vi "eta2cont (SubVI).vi"(11 "eta_disc":dbl[](array[numeric])) -> (2 "count":dbl, 3 "eta_cont":dbl[](array[numeric]))   [LabVIEW 2014]
uses:
  <vilib>/imath/engines/lvmath2/RunTimeEngine/IndexRead/NIMS V(S).vi
  <instcachedir>/0/NIMS V(S)_0488751826AF41519A22953C041130DC.lvgen/NIMS V(S)_0488751826AF41519A22953C041130DC_000.vi
  <vilib>/imathl/engines/lvmath/Functions/Error Handling/Create Error.vi
  <vilib>/imath/engines/lvmath2/RunTimeEngine/IndexReplace/NIMS V(S)=S.vi
  <instcachedir>/0/NIMS V(S)=S_2D52C4EC15D8415E870AEE69FB516CCA.lvgen/NIMS V(S)=S_2D52C4EC15D8415E870AEE69FB516CCA_000.vi
  <vilib>/imath/engines/lvmath2/RunTimeEngine/NodeEndStatement/NIMS_NodeEndStatement_Output.vi
  <instcachedir>/0/NIMS_NodeEndStatement_Output_53EC0D466D134D7ABD903AC30B43404B.lvgen/NIMS_NodeEndStatement_Output_53EC0D466D134D7ABD903AC30B43404B_005.vi
  <instcachedir>/0/NIMS_NodeEndStatement_Output_53EC0D466D134D7ABD903AC30B43404B.lvgen/NIMS_NodeEndStatement_Output_53EC0D466D134D7ABD903AC30B43404B_001.vi
  <vilib>/imath/engines/lvmath2/RunTimeEngine/ErrorHandling/NIMS_Finalize Error.vi
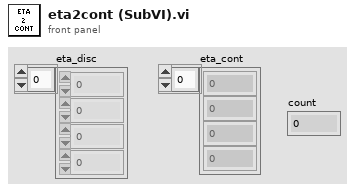
[diagram p1: front panel]
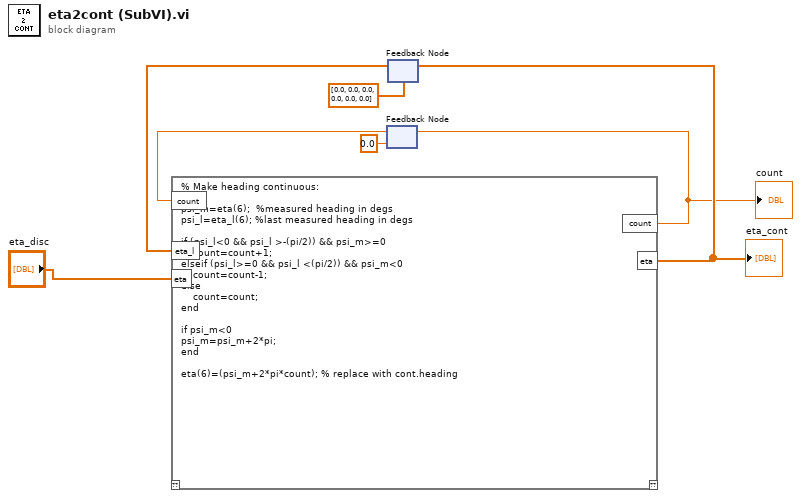
[diagram p0: block diagram]
diagram:
  n1 = feedback #1(0.0 ("count")) -> (w4:dbl)
  n2 = feedback #2(dbl[] [0.0, 0.0, 0.0, 0.0, 0.0, 0.0] ("eta")) -> (w6:dbl[])
  n3 = mathscript code="% Make heading continuous:\n\npsi_m=eta(6);  %measured heading in degs\npsi_l=eta_l(6); %last measured heading in degs\n\nif (psi_l<0 && psi_l >-(pi/2)) && psi_m>=0\n    count=count+1;    \nelseif (psi_l>=0 && psi_l <(pi/2)) && psi_m<0\n    count=count-1;\nelse    \n    count=count;\nend\n\nif psi_m<0\npsi_m=psi_m+2*pi;\nend\n\neta(6)=(psi_m+2*pi*count); % replace with cont.heading"("eta"="eta_disc", "eta_l"=w6, "count"=w4) -> ("count"=w3:dbl, "eta"=w5:dbl[])  [unwired: 1 in, 1 out]
  "eta_cont" <- w5
  "count" <- w3
  n4 = feedback-in #1(w3) -> ()
  n5 = feedback-in #2(w5) -> ()
